vi "서보모터 _속도제어.vi"() -> ()   [LabVIEW 2014]
uses:
  <vilib>/DAQmx/create/channels.llb/DAQmx Create Channel (CO-Pulse Generation-Frequency).vi
  <vilib>/DAQmx/configure/timing.llb/DAQmx Timing (Implicit).vi
  <vilib>/DAQmx/write.llb/DAQmx Write (Counter Frequency 1Chan 1Samp).vi
panel:
  in  "frequency":dbl=50.0 format="%.6f"
  in  "정지":bool
  in  "counter":tag="cDAQ3Mod1/ctr0" caption="카운터"
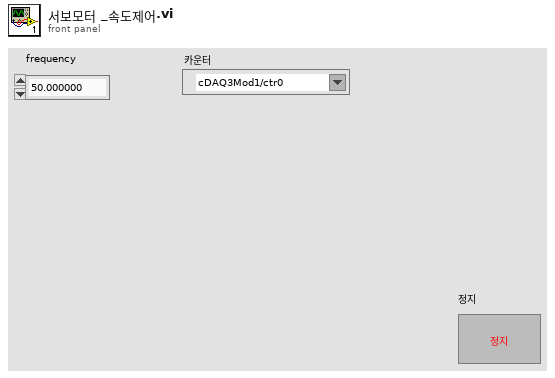
[diagram p1: front panel]
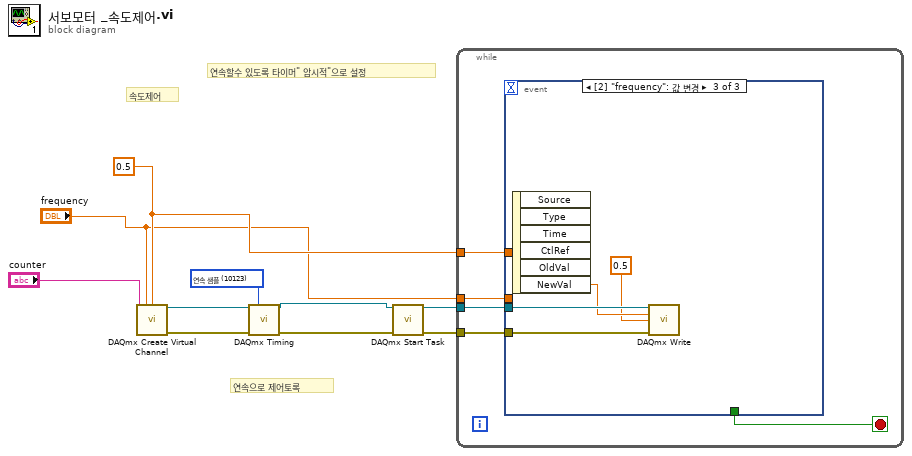
[diagram p0: block diagram]
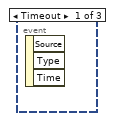
[diagram p2: hidden frame]
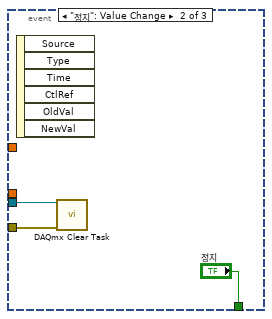
[diagram p3: hidden frame]
diagram:
  w3 = 0.5 ("duty cycle")
  w9 = 10123 items=["유한 샘플"=10178, "연속 샘플"=10123, "하드웨어 타이밍에 의한 단일 포인트"=12522] ("sample mode")
  # "속도제어"
  # "연속으로 제어토록"
  # "연속할수 있도록 타이머\" 암시적\"으로 설정"
  n1 = call-poly <vilib>:"DAQmx Create Virtual Channel.vi"("frequency"="frequency", "duty cycle"=w3, "counter"="counter") -> ("task out"=w1:refnum<k21>, "error out"=w7:errorcluster)  [unwired: 11 in]
  n2 = call-poly <vilib>:"DAQmx Timing.vi"("task/channels in"=w1, "sample mode"=w9, "error in"=w7) -> ("task out"=w8:refnum<k21>, "error out"=w6:errorcluster)  [unwired: 11 in]
  n3 = call <vilib>:"DAQmx Start Task.vi"("task/channels in"=w8, "error in"=w6) -> ("task out"=w5:refnum<k21>, "error out"=w4:errorcluster)  [unwired: 12 in]
  n4 = while {
    tunnel: w5 -> [w15]
    tunnel: w4 -> [w14]
    tunnel: w3 -> [w12]
    tunnel: "frequency" -> [w11]
    stop <- w13 stop-if-true
    n5 = event shown="[2] \"frequency\": 값 변경" {
      selector: _ -> [_ _ _]
      dyn-events: _ -> [_ _ _]
      timeout: _ -> [_ _ _]
      tunnel: w15 -> [_ w18 w22]
      tunnel: w14 -> [_ w17 w21]
      tunnel: [_ "정지" _] -> w13
      tunnel: w12 -> [_ _ _]
      tunnel: w11 -> [_ _ _]
      event Timeout {
        n6 = event-data() -> ()  [unwired: 1 in, 3 out]
      }
      event "정지": Value Change {
        n7 = event-data() -> ()  [unwired: 1 in, 6 out]
        n8 = call <vilib>:"DAQmx Clear Task.vi"("task in"=w18, "error in"=w17) -> ()  [unwired: 13 in, 1 out]
      }
      event "frequency": Value Change {
        n9 = event-data() -> ("NewVal"=w20:dbl)  [unwired: 1 in, 5 out]
        n10 = call-poly <vilib>:"DAQmx Write.vi"("task/channels in"=w22, "frequency"=w20, "duty cycle"=0.5 ("frequency"), "error in"=w21) -> ()  [unwired: 9 in, 3 out]
      }
    }
  }
